vi "Configure Local Node Characteristics.vi"(0 "VISA resource name":refnum<visa-resource-name>, 1 "Power Frequency (0: 60 Hz)":i32(ring) items=["60 Hz", "50 Hz"], 2 "Auto Output Error Message (F: Disable)":bool, 5 "Auto Detect Power Frequency (T: Enable)":bool=TRUE, 7 "Enable IEEE488.2 Command Prompt (T: Enable)":bool=TRUE, 9 "Password Mode (0: None)":i32(ring) items=["None", "Web Interface", "LAN Interface", " ALL Interface"], 11 "error in (no error)":errorcluster, 12 "Password":string) -> (4 "VISA resource name out":refnum<visa-resource-name>, 15 "error out":errorcluster)   [LabVIEW 2017, in "Keithley 2600 Series.lvlib"]
doc: "Configures the basic settings of the instrument."
uses:
  <instrlib>/Keithley 2600 Series/Keithley 2600 Series.lvlib
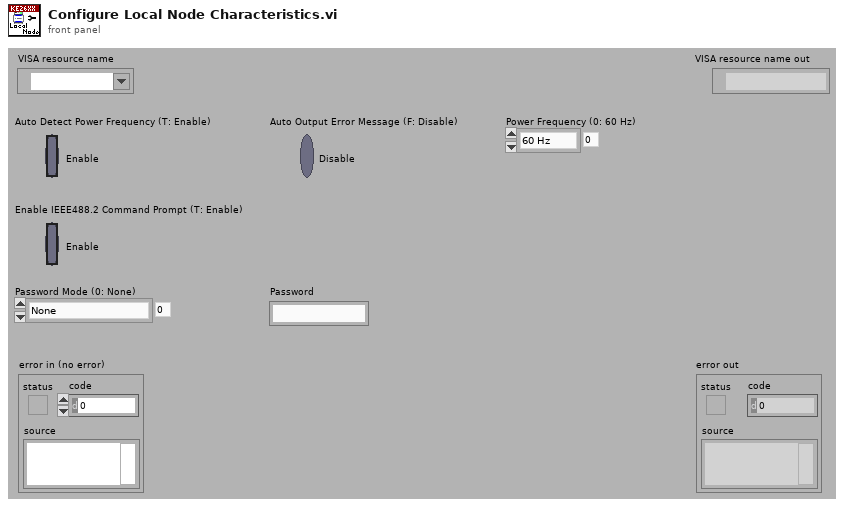
[diagram p1: front panel]
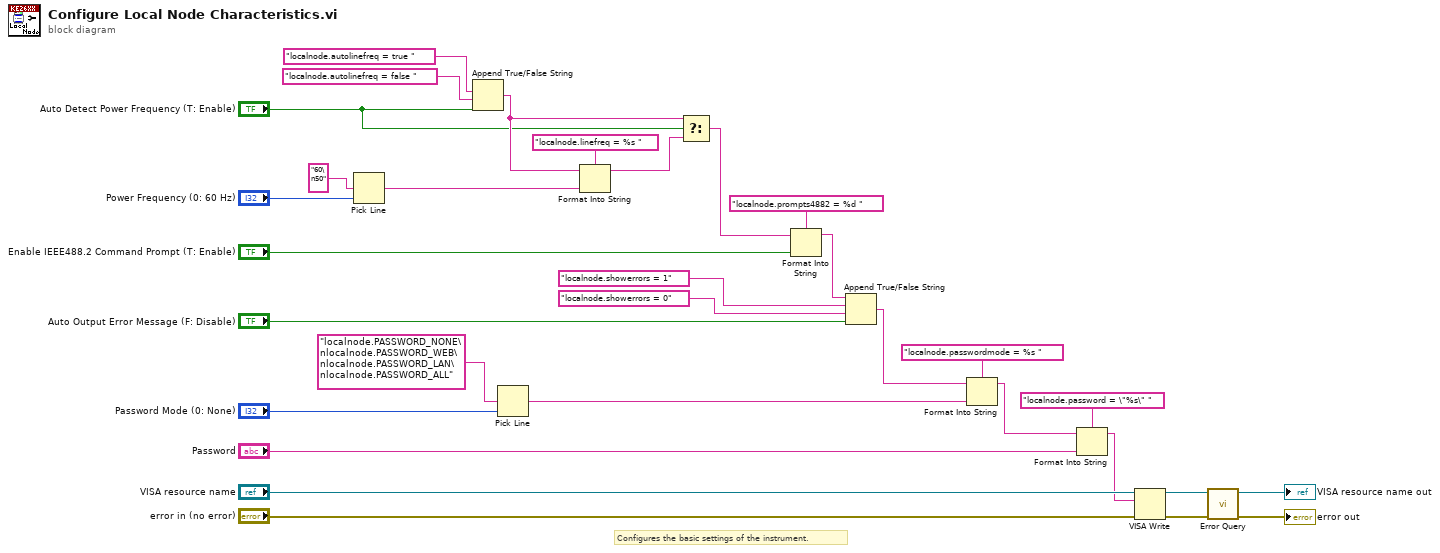
[diagram p0: block diagram]
diagram:
  # "Configures the basic settings of the instrument."
  n1 = Pick Line(multi-line string="60\n50", line index="Power Frequency (0: 60 Hz)") -> (output string=w23:string)  [unwired: 1 in]
  n2 = Append True/False String(1:"Auto Detect Power Frequency (T: Enable)", 2:"localnode.autolinefreq = false ", 3:"localnode.autolinefreq = true ") -> (0:w22:string)  [unwired: 1 in]
  n3 = Pick Line(multi-line string="localnode.PASSWORD_NONE\nlocalnode.PASSWORD_WEB\nlocalnode.PASSWORD_LAN\nlocalnode.PASSWORD_ALL", line index="Password Mode (0: None)") -> (output string=w9:string)  [unwired: 1 in]
  n4 = Format Into String(format string="localnode.linefreq = %s ", initial string=w22, w23) -> (resulting string=w21:string)  [unwired: 1 in, 1 out]
  n5 = Select(t=w22, s="Auto Detect Power Frequency (T: Enable)", f=w21) -> (s? t:f=w19:string)
  n6 = Format Into String(format string="localnode.prompts4882 = %d ", initial string=w19, "Enable IEEE488.2 Command Prompt (T: Enable)") -> (resulting string=w15:string)  [unwired: 1 in, 1 out]
  n7 = Append True/False String(1:"Auto Output Error Message (F: Disable)", 2:"localnode.showerrors = 0", 3:"localnode.showerrors = 1", 4:w15) -> (0:w6:string)
  n8 = Format Into String(format string="localnode.passwordmode = %s ", initial string=w6, w9) -> (resulting string=w7:string)  [unwired: 1 in, 1 out]
  n9 = Format Into String(format string="localnode.password = \"%s\" ", initial string=w7, "Password") -> (resulting string=w5:string)  [unwired: 1 in, 1 out]
  n10 = VISA Write(VISA resource name="VISA resource name", write buffer=w5, error in (no error)="error in (no error)") -> (VISA resource name out=w27:refnum<visa-resource-name>, error out=w3:errorcluster)  [unwired: 1 out]
  n11 = call <instrlib>:"Error Query.vi"("error in (no error)"=w3, "VISA resource name"=w27) -> ("error out"=→"error out":errorcluster, "VISA resource name out"=→"VISA resource name out":refnum<visa-resource-name>)  [unwired: 6 in, 2 out]
